vi "Format Child Text.vi"(10 "Type":string, 11 "Value":string) -> (3 "Child Text":string[](array[string]))   [LabVIEW 2019, in "BlueVariantView.lvlib"]
uses:
  BlueVariantView.lvlib
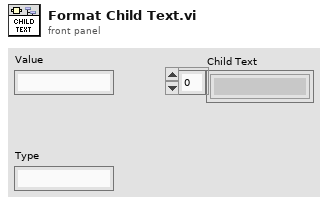
[diagram p1: front panel]
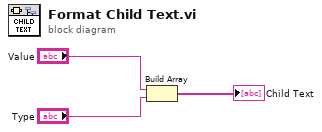
[diagram p0: block diagram]
diagram:
  n1 = Build Array("Value", "Type") -> (→"Child Text":string[])
